vi "NICAN_CAN_Transmit.vi"() -> ()   [LabVIEW 2018]
doc: "Demonstrates how to transmit multiple CAN frames via the Network Interface.\n\nTo transmit frames:\n- select the CAN Network Interface (i.e. CAN0, CAN1, etc.)\n-select the Frame Type (Start Trigger, Data, Delay)- refer to the manual \n- select the Baud Rate\n- select the Arbitration ID\n-run the VI\n\nThe VI transmits multiple CAN frame, each time the WRITE button is pressed. The values for the Data Length, the Data and the RTR flag can be changed for each single Frame.\n\n-press STOP to abort the VI"
uses:
  <vilib>/nican/nican.llb/CanFrameTimed.ctl
  <vilib>/nican/nican.llb/ncNetAttr.ctl
panel:
  in  "Timestamped Transmit? (PCI/PXI/PCMCIA only)":bool
  in  "Interface":string(combo)="CAN1"
  in  "Data":T1[](array[typedef])=[{"Timestamp"=0.0, "ArbitrationId"=5, "IsRemote"=0, "DataLength"=8, "Data"=[0, 0, 0, 0, 0, 0, 0, 0]}, {"Timestamp"=0.01, "ArbitrationId"=5, "IsRemote"=0, "DataLength"=8, "Data"=[1, 1, 1, 1, 1, 1, 1, 1]}, {"Timestamp"=0.02, "ArbitrationId"=5, "IsRemote"=0, "DataLength"=8, "Data"=[2, 2, 2, 2, 2, 2, 2, 2]}, {"Timestamp"=0.03, "ArbitrationId"=5, "IsRemote"=0, "DataLength"=8, "Data"=[3, 3, 3, 3, 3, 3, 3, 3]}, {"Timestamp"=0.04, "ArbitrationId"=5, "IsRemote"=0, "DataLength"=8, "Data"=[4, 4, 4, 4, 4, 4, 4, 4]}, {"Timestamp"=1.0, "ArbitrationId"=5, "IsRemote"=0, "DataLength"=8, "Data"=[5, 5, 5, 5, 5, 5, 5, 5]}] {"Data" format="%.0x"; "ArbitrationId" format="%.0x"; "Timestamp" format="%<%H:%M:%S%3u>t"}
  in  "Number to Write":u32=6
  in  "Write frames":bool
  in  "Baudrate":u32=125000
  in  "stop":bool
  # "See VI Info <Ctrl+I> for more information on how to use this example"
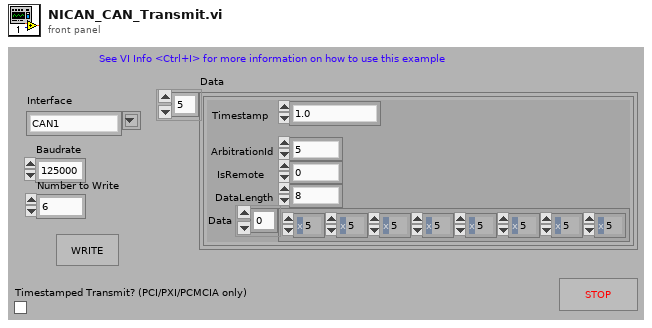
[diagram p1: front panel]
types:
  T1 = typedef "CanFrameTimed.ctl" = cluster{"Timestamp":dbl, "ArbitrationId":u32, "IsRemote":u8, "DataLength":u8, "Data":u8[]}
  T2 = typedef "ncNetAttr.ctl" = cluster{"Start On Open":enum32{"FALSE", "TRUE"}, "Baud Rate":u32, "Read Queue Length":u32, "Write Queue Length":u32, "Standard Comparator":u32, "Standard Mask":u32, "Extended Comparator":u32, "Extended Mask":u32}
  T3 = typedef "xobjhandle.ctl" = u32
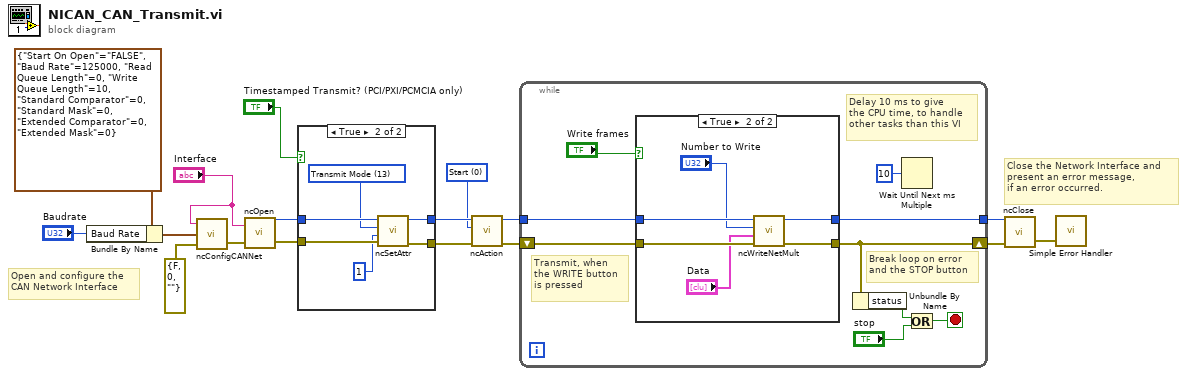
[diagram p0: block diagram]
diagram:
  w3 = u32 0 items=["Start", "Stop", "Reset", "Output on RTSI line"] ("Opcode")
  # "Open and configure the \nCAN Network Interface"
  # "Close the Network Interface and \npresent an error message, \nif an error occurred."
  n1 = Bundle By Name(cluster=T2 {"Start On Open"=enum."FALSE", "Baud Rate"=125000, "Read Queue Length"=0, "Write Queue Length"=10, "Standard Comparator"=0, "Standard Mask"=0, "Extended Comparator"=0, "Extended Mask"=0} ("CAN Network Interface Config"), "Baud Rate"="Baudrate") -> (w14:T2)
  n2 = call <vilib>:"ncConfigCANNet.vi"("Error in"=errorcluster {"status"=FALSE, "code"=0, "source"=""}, "CAN Network Interface Config"=w14, "ObjName"="Interface") -> ("Error out"=w16:errorcluster)  [unwired: 2 in]
  n3 = call <vilib>:"ncOpen.vi"("Error in"=w16, "ObjName"="Interface") -> ("Error out"=w9:errorcluster, "ObjHandle out"=w8:T3)
  n4 = case shown="True" "Timestamped Transmit? (PCI/PXI/PCMCIA only)" {
    tunnel: w9 -> [w18 w25]
    tunnel: w8 -> [w19 w24]
    tunnel: [w18 w21] -> w7
    tunnel: [w19 w20] -> w6
    frame False {
    }
    frame True {
      w23 = u32 13 items=["ReadMult Size for Notification", "User RTSI Frame", "Log Comm Warnings", "Listen Only?", "Self Reception?", "Single Shot Transmit?", "Series 2 Filter Mode", "Series 2 Mask", "Series 2 Comparator", "Transceiver Type", "Transceiver Mode", "Transceiver External Outputs", "(reserved)", "Transmit Mode", "Log Start Trigger?", "Timestamp Format", "Master Timebase Rate", "Virtual Bus Timing", "Timeline Recovery"] ("AttrId")
      n5 = call <vilib>:"ncSetAttr.vi"("Error in"=w25, "AttrValue"=u32 1, "AttrId"=w23, "ObjHandle in"=w24) -> ("Error out"=w21:errorcluster, "ObjHandle out"=w20:T3)
    }
  }
  n6 = call <vilib>:"ncAction.vi"("Error in"=w7, "Opcode"=w3, "ObjHandle in"=w6) -> ("Error out"=w4:errorcluster, "ObjHandle out"=w5:T3)  [unwired: 1 in]
  n7 = while {
    shift-left: w4 -> [w27]
    shift-right: [w26] -> w11
    tunnel: w5 -> [w29]
    tunnel: [w33] -> w12
    stop <- w30 stop-if-true
    # "Transmit, when\nthe WRITE button \nis pressed"
    # "Delay 10 ms to give \nthe CPU time, to handle \nother tasks than this VI"
    # "Break loop on error \nand the STOP button"
    n8 = case shown="True" "Write frames" {
      tunnel: w29 -> [w35 w41]
      tunnel: w27 -> [w36 w42]
      tunnel: [w36 w40] -> w26
      tunnel: [w35 w39] -> w33
      frame False {
      }
      frame True {
        n9 = call <vilib>:"ncWriteNetMult.vi"("Error in"=w42, "Data"="Data", "Number to Write"="Number to Write", "ObjHandle in"=w41) -> ("Error out"=w40:errorcluster, "ObjHandle out"=w39:T3)  [unwired: 6 in]
      }
    }
    n10 = Unbundle By Name(w26) -> ("status"=w32:bool)
    n11 = Wait Until Next ms Multiple(millisecond multiple=u32 10) -> ()  [unwired: 1 out]
    n12 = Or(x=w32, y="stop") -> (x .or. y?=w30:bool)
  }
  n13 = call <vilib>:"ncClose.vi"("Error in"=w11, "ObjHandle in"=w12) -> ("Error out"=w17:errorcluster)  [unwired: 1 in]
  n14 = call <vilib>:"Simple Error Handler.vi"("error in (no error)"=w17) -> ()  [unwired: 4 in, 5 out]
